vi "Configure Source Real Time Eye.vi"(6 "UI Scale (0.25)":dbl=0.25, 7 "Waveform Source (0: Channel 1)":i32(ring) items=["Channel 1", "Channel 2", "Channel 3", "Channel 4", "Common 1", "Common 2", "Differential 1", "Differential 2", "Memory 1", "Memory 2", "Memory 3", "Memory 4", "Function 1", "Function 2", "Function 3", "Function 4", "Function 5", "Function 6", "Function 7", "Function 8", "Function 9", "Function 10", "Function 11", "Function 12", "Function 13", "Function 14", "Function 15", "Function 16"], 8 "error in (no error)":errorcluster, 9 "UI Position (0)":dbl, 10 "Enable Real Time Eye (F: Disable)":bool, 11 "VISA resource name":refnum<visa-resource-name>) -> (0 "error out":errorcluster, 3 "VISA resource name out":refnum<visa-resource-name>)   [LabVIEW 2020, in "Agilent 90000 Series.lvlib"]
doc: "Configures the real time eye parameters (with source).\n\n<b>Note:</b> \nThis VI is new in firmware version 4.50."
uses:
  Agilent 90000 Series.lvlib
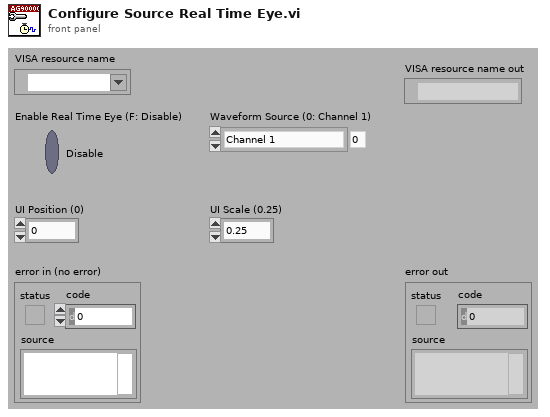
[diagram p1: front panel]
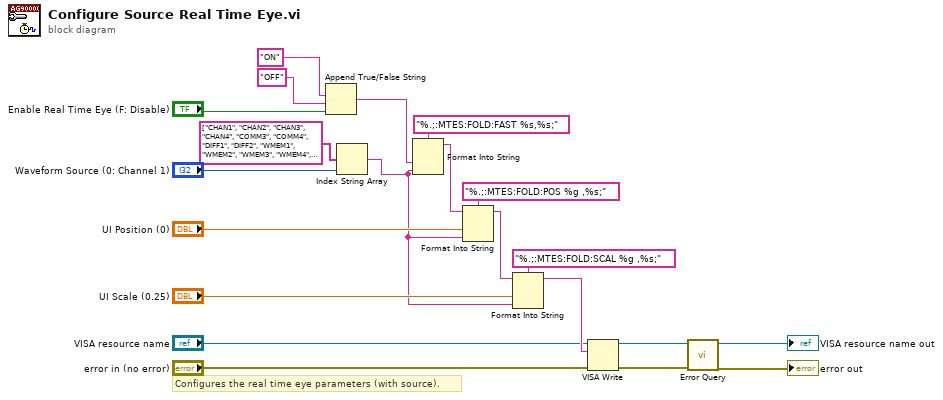
[diagram p0: block diagram]
diagram:
  # "Configures the real time eye parameters (with source)."
  n1 = Append True/False String(1:"Enable Real Time Eye (F: Disable)", 2:"OFF", 3:"ON") -> (0:w17:string)  [unwired: 1 in]
  n2 = Index String Array(1:"Waveform Source (0: Channel 1)", 2:string[] ["CHAN1", "CHAN2", "CHAN3", "CHAN4", "COMM3", "COMM4", "DIFF1", "DIFF2", "WMEM1", "WMEM2", "WMEM3", "WMEM4", "FUNC1", "FUNC2", "FUNC3", "FUNC4", "FUNC5", "FUNC6", "FUNC7", "FUNC8", "FUNC9", "FUNC10", "FUNC11", "FUNC12", "FUNC13", "FUNC14", "FUNC15", "FUNC16"] ("string array")) -> (0:w2:string)  [unwired: 1 in]
  n3 = Format Into String(format string="%.;:MTES:FOLD:FAST %s,%s;", w17, w2) -> (resulting string=w16:string)  [unwired: 2 in, 1 out]
  n4 = Format Into String(format string="%.;:MTES:FOLD:POS %g ,%s;", initial string=w16, "UI Position (0)", w2) -> (resulting string=w13:string)  [unwired: 1 in, 1 out]
  n5 = Format Into String(format string="%.;:MTES:FOLD:SCAL %g ,%s;", initial string=w13, "UI Scale (0.25)", w2) -> (resulting string=w10:string)  [unwired: 1 in, 1 out]
  n6 = VISA Write(VISA resource name="VISA resource name", write buffer=w10, error in (no error)="error in (no error)") -> (VISA resource name out=w7:refnum<visa-resource-name>, error out=w6:errorcluster)  [unwired: 1 out]
  n7 = call "Error Query.vi"("error in (no error)"=w6, "VISA resource name"=w7) -> ("error out"=→"error out":errorcluster, "VISA resource name out"=→"VISA resource name out":refnum<visa-resource-name>)  [unwired: 6 in, 2 out]
